vi "02guarda_config_equipos.vi"(1 "Nº equipo":i32, 2 "Config equipo":T1={"Modelo"="", "IP "="", "Puerto:"=0, "Time Out"=0, "Med Princ"=0, "Time sin rx"=0, "Reintento"=0, "Ref PD"=200} {"Ref PD" max=10000 step=1}, 3 "exe path":string) -> ()   [LabVIEW 2010]
uses:
  <vilib>/Utility/file.llb/Write To Spreadsheet File (string).vi
  <vilib>/Utility/file.llb/Write To Spreadsheet File (I64).vi
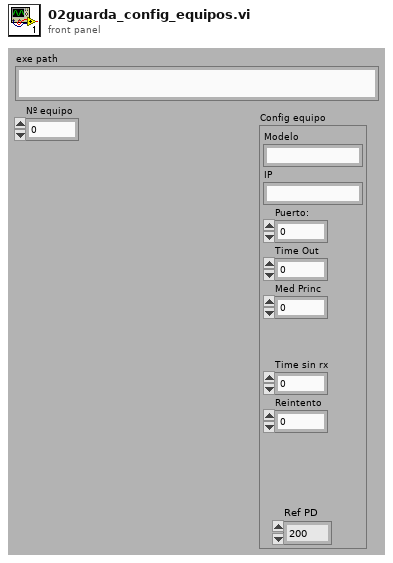
[diagram p1: front panel]
types:
  T1 = cluster{"Modelo":string, "IP ":string, "Puerto:":u16, "Time Out":u16, "Med Princ":u16, "Time sin rx":u16, "Reintento":u16, "Ref PD":u16}
  T2 = cluster{"Puerto:":u16, "Time Out":u16, "Med Princ":u16, "Time sin rx":u16, "Reintento":u16, "Ref PD":u16}
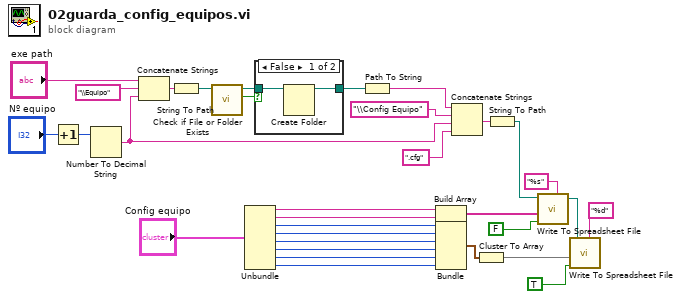
[diagram p0: block diagram]
diagram:
  n1 = Increment(x="Nº equipo") -> (x+1=w12:i32)
  n2 = Number To Decimal String(number=w12) -> (decimal integer string=w29:string)  [unwired: 1 out]
  n3 = Concatenate Strings("exe path", "\\Equipo" ("replace string (\"\")"), w29) -> (w26:string)
  n4 = String To Path(string=w26) -> (path=w25:path)
  n5 = call <vilib>:"Check if File or Folder Exists.vi"("path"=w25) -> ("file or folder exists?"=w24:bool, "dup path"=w23:path)  [unwired: 1 in, 8 out]
  n6 = Unbundle("Config equipo") -> ("Modelo"=w4:string, "IP"=w5:string, "Puerto:"=w6:u16, "Time Out"=w7:u16, "Med Princ"=w8:u16, "Time sin rx"=w9:u16, "Reintento"=w10:u16, "Ref PD"=w11:u16)
  n7 = case shown="False" w24 {
    tunnel: [w34 w35] -> w32
    tunnel: w23 -> [w33 w35]
    frame False {
      n8 = Create Folder(path (use dialog)=w33) -> (created path=w34:path)  [unwired: 1 in, 3 out]
    }
    frame True {
    }
  }
  n9 = Path To String(path=w32) -> (string=w3:string)
  n10 = Build Array(w4, w5) -> (w15:string[])
  n11 = Bundle("Puerto:"=w6, "Time Out"=w7, "Med Princ"=w8, "Time sin rx"=w9, "Reintento"=w10, "Ref PD"=w11) -> (w14:T2)  [unwired: 1 out]
  n12 = Concatenate Strings(w3, "\\Config Equipo" ("replace string (\"\")"), w29, ".cfg" ("replace string (\"\")")) -> (w31:string)
  n13 = Cluster To Array(cluster=w14) -> (array=w17:u16[])
  n14 = String To Path(string=w31) -> (path=w16:path)
  n15 = call-poly <vilib>:"Write To Spreadsheet File.vi"("format (%s)"="%s" ("format (%d)"), "append to file? (new file:F)"=FALSE, "1D data"=w15, "file path (dialog if empty)"=w16) -> ("new file path (Not A Path if cancelled)"=w20:path)  [unwired: 2 in, 2 out]
  n16 = call-poly <vilib>:"Write To Spreadsheet File.vi"("format (%d)"="%d", "append to file? (new file:F)"=TRUE, "1D data"=w17, "file path (dialog if empty)"=w20) -> ()  [unwired: 2 in, 3 out]
